vi "Main.vi"(8 "error in (no error)":errorcluster) -> ()   [LabVIEW 2017, in "FlagImpairModule.lvlib"]
uses:
  FlagImpairModule.lvlib
  <userlib>/NIST/ModuleAdminLib/ModuleAdmin/ModuleAdmin.lvclass
  C:/Program Files (x86)/National Instruments/LabVIEW 2017/user.lib/NIST/ModuleAdminLib/ModuleAdminBase/ModuleAdminBase.lvclass
  PublicAPI/Arguments/Requests/clStopArgument.ctl
  FlagImpairPlugins/FlagImpairPluginBase_class/FlagImpairPluginBase.lvclass
  C:/Program Files (x86)/National Instruments/LabVIEW 2017/user.lib/NIST/BaseClasses/BasePlugin_class/BasePlugin.lvclass
  <userlib>/NIST/ModuleAdminLib/ModuleAdmin/ModuleAdmin.lvclass/ModuleAdmin.ctl
  <userlib>/NIST/BaseClasses/BasePlugin_class/BasePlugin.lvclass/BasePlugin.ctl
  PublicAPI/Arguments/Requests/clFlagImpairConfig.ctl
  FlagImpairPlugins/FlagImpairPluginBase_class/TypeDefs/clFlagImpairConfig.ctl
  PublicAPI/Arguments/Requests/dblFlagImpairParams.ctl
  PublicAPI/Arguments/Requests/dblTimeArray.ctl
  <vilib>/Utility/error.llb/DialogType.ctl
  <userlib>/NIST/ModuleAdminLib/ModuleAdmin/Accessors/Read ShowPanel_.vi
  <userlib>/NIST/ModuleAdminLib/ModuleAdmin/Accessors/Write ShowPanel_.vi
  <userlib>/NIST/BaseClasses/BasePlugin_class/Accessors/Write PluginIniFilePath.vi
  <userlib>/NIST/BaseClasses/BasePlugin_class/Accessors/Read PluginIniFilePath.vi
  <userlib>/NIST/ModuleAdminLib/ModuleAdmin/Accessors/Read CloneRegRef.vi
  <vilib>/Utility/error.llb/Error Cluster From Error Code.vi
  FlagImpairPlugins/FlagImpairPluginBase_class/Accessors/Write clFlagImpairConfig.vi
  FlagImpairPlugins/FlagImpairPluginBase_class/Accessors/Read clFlagImpairConfig.vi
  FlagImpairPlugins/FlagImpairPluginBase_class/Accessors/Write FlagImpairParams.vi
  FlagImpairPlugins/FlagImpairPluginBase_class/Accessors/Read FlagImpairParams.vi
  FlagImpairPlugins/FlagImpairPluginBase_class/Accessors/Write TimeArray.vi
  FlagImpairPlugins/FlagImpairPluginBase_class/Accessors/Read TimeArray.vi
  FlagImpairPlugins/FlagImpairPluginBase_class/Accessors/Get FlagImpairmentArray.vi
  <vilib>/ErrorRing/Error Ring.xnode
  <userlib>/NIST/ModuleAdminLib/CloneRegistration/CloneRegistration.lvclass
  <userlib>/NIST/ModuleAdminLib/ModuleAdmin.lvlib
  <userlib>/NIST/BaseClasses/Object_class/BaseObject.lvclass
panel:
  out "error out":errorcluster
  in  "ModuleAdmin":refnum<class "ModuleAdmin.lvclass">
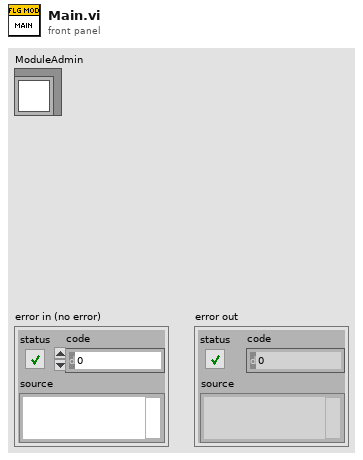
[diagram p1: front panel]
types:
  T1 = typedef "FlagImpairModule.lvlib/clRequestEvents.ctl" = cluster{"StopRequest":refnum<user-event>, "WriteFlagImpairConfigRequest":refnum<user-event>, "ReadFlagImpairConfigRequest":refnum<user-event>, "WriteFlagImpairParamsRequest":refnum<user-event>, "ReadFlagImpairParamsRequest":refnum<user-event>, "WriteTimeArrayRequest":refnum<user-event>, "ReadTimeArrayRequest":refnum<user-event>, "GetFlagImpairmentRequest":refnum<user-event>, "LoadPluginRequest":refnum<user-event>, "ReadPluginPathRequest":refnum<user-event>, "ShowPanelRequest":refnum<user-event>}
  T2 = typedef "FlagImpairModule.lvlib/clBroadcastEvents.ctl" = cluster{"DidInit":refnum<user-event>, "StatusUpdate":refnum<user-event>, "ErrorReport":refnum<user-event>, "DidStop":refnum<user-event>, "ReadFlagImpairConfig":refnum<user-event>, "ReadPluginINIFilePath":refnum<user-event>, "ReadFlagImpairParams":refnum<user-event>, "ReadTimeArray":refnum<user-event>, "GetFlagImpairment":refnum<user-event>}
  T3 = typedef "FlagImpairModule.lvlib/clStopArgument.ctl" = cluster{"Exit via Stop Module Req?":bool, "Wait for Module to stop?":bool, "ModuleAdmin":refnum<class "ModuleAdmin.lvclass">}
  T4 = enum32{"Invalid", "Standard", "Closed", "Hidden", "Minimized", "Maximized"}
  T5 = typedef "FlagImpairPlugins.lvlib/FlagImpairPluginBase.lvclass/clFlagImpairConfig.ctl" = cluster{"FlagImpairmentType":u16}
  T6 = typedef "FlagImpairModule.lvlib/clFlagImpairConfig.ctl" = cluster{"FlagImpairmentType":u16}
  T7 = typedef "FlagImpairModule.lvlib/dblFlagImpairParams.ctl" = dbl[][]
  T8 = typedef "FlagImpairModule.lvlib/dblTimeArray.ctl" = dbl[]
  T9 = typedef "FlagImpairPlugins.lvlib/FlagImpairPluginBase.lvclass/FlagImpairmentArray.ctl" = u32[]
  T10 = typedef "DialogType.ctl" = u16
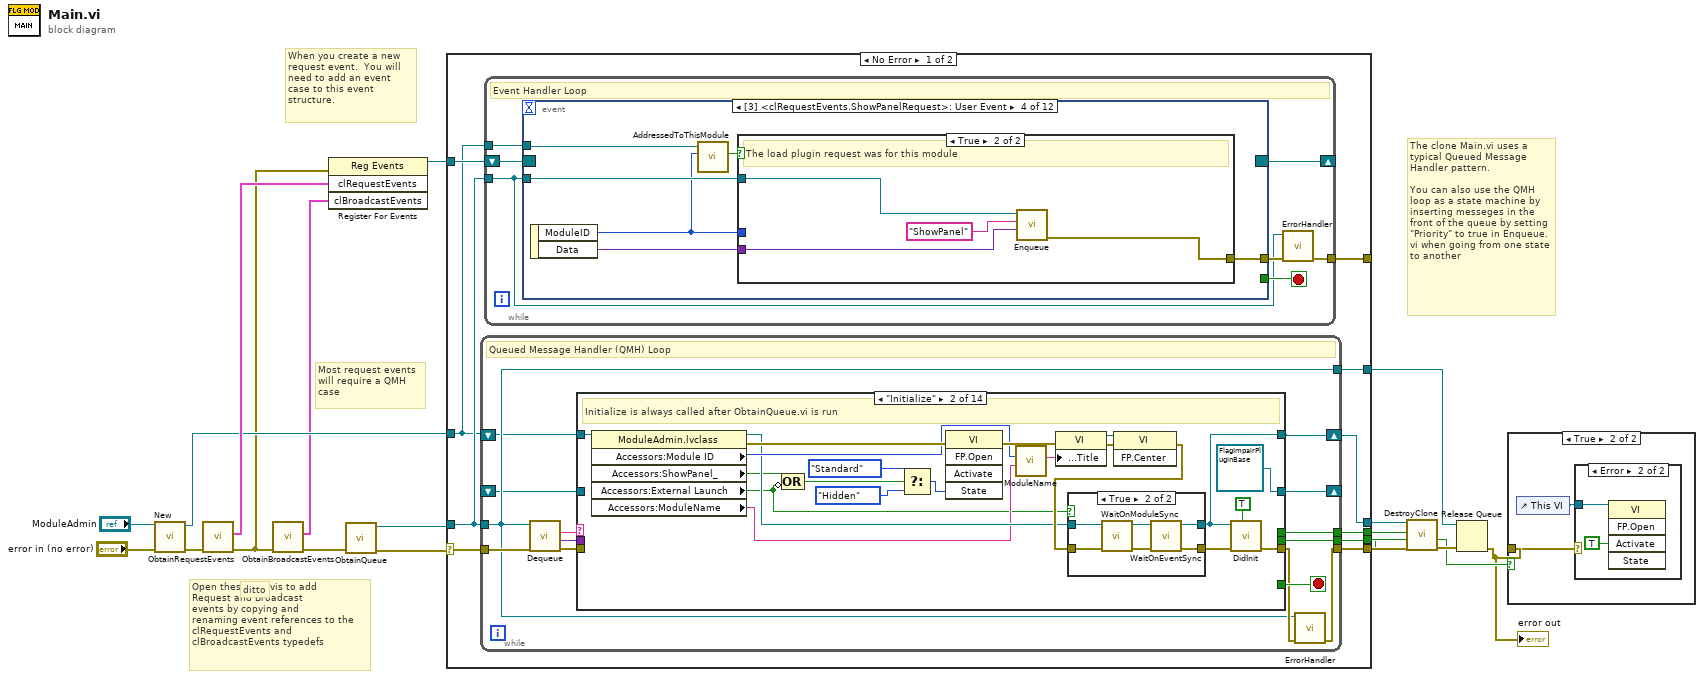
[diagram p0: block diagram]
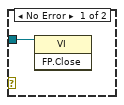
[diagram p3: hidden frame]
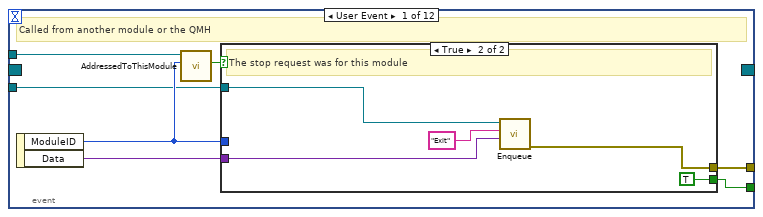
[diagram p4: hidden frame]
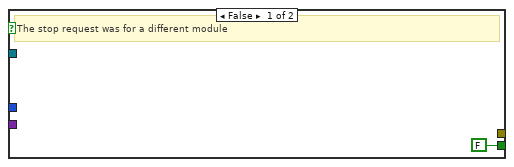
[diagram p5: hidden frame]
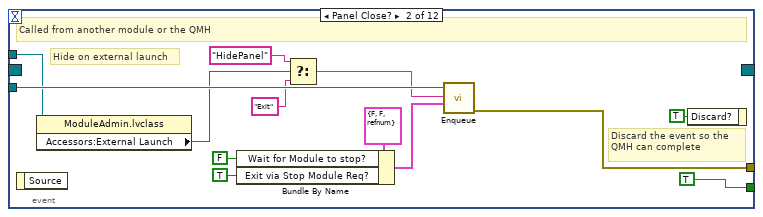
[diagram p6: hidden frame]
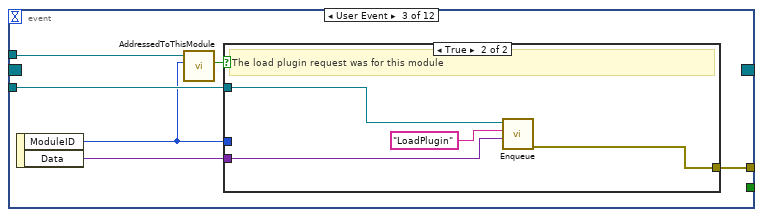
[diagram p7: hidden frame]
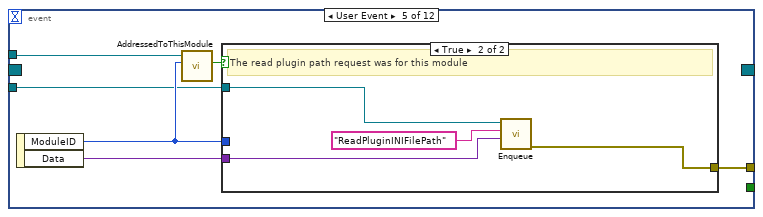
[diagram p10: hidden frame]
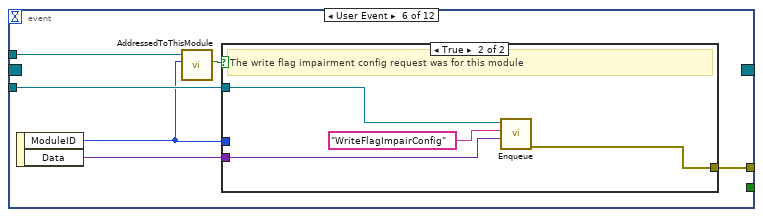
[diagram p12: hidden frame]
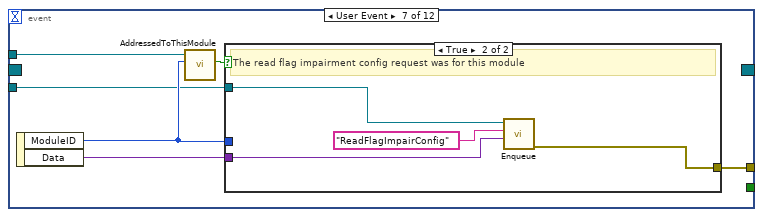
[diagram p14: hidden frame]
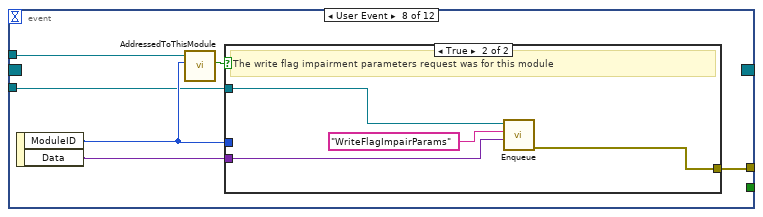
[diagram p16: hidden frame]
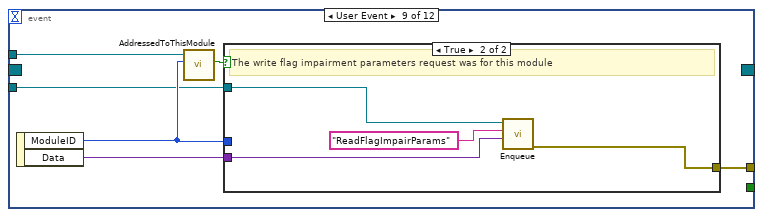
[diagram p18: hidden frame]
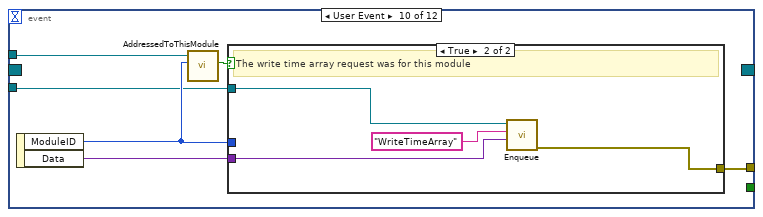
[diagram p20: hidden frame]
diagram:
  # "The clone Main.vi uses a typical Queued Message Handler pattern.  \n\nYou can also use the QMH loop as a state machine by inserting messeges in the front of the queue by setting \"Priority\" to true in Enqueue.vi when going from one state to another"
  # "Open these two vis to add\nRequest and Broadcast \nevents by copying and \nrenaming event references to the \nclRequestEvents and \nclBroadcastEvents typedefs"
  # "ditto"
  # "Most request events\nwill require a QMH\ncase"
  # "When you create a new request event.  You will need to add an event case to this event structure."
  n1 = call <userlib>:"New.vi"("error in (no error)"="error in (no error)", "ModuleAdmin"="ModuleAdmin") -> ("error out"=w17:errorcluster, "ModuleAdmin"=w13:refnum<class "ModuleAdmin.lvclass">)  [unwired: 7 in, 1 out]
  n2 = call "ObtainRequestEvents.vi"("error in (no error)"=w17) -> ("error out"=w10:errorcluster, "clRequestEvents"=w16:T1)  [unwired: 9 in]
  n3 = call "ObtainBroadcastEvents.vi"("error in (no error)"=w10) -> ("error out"=w11:errorcluster, "clBroadcastEvents"=w9:T2)  [unwired: 9 in]
  n4 = register-events(error in=w10, w16, w9) -> (reference out=w8:refnum<event-registration>)  [unwired: 1 in, 1 out]
  n5 = call "ObtainQueue.vi"("error in (no error)"=w11) -> ("error out"=w15:errorcluster, "MessageQueue"=w14:refnum<queue>)  [unwired: 9 in]
  n6 = case shown="No Error" w15 {
    selector: w15 -> [w29 w407]
    tunnel: w14 -> [w27 w403]
    tunnel: w13 -> [w24 w404]
    tunnel: [w28 w405] -> w7
    tunnel: [w26 w403] -> w12
    tunnel: w8 -> [w25 _]
    tunnel: [w23 w402] -> w5
    tunnel: [w22 _] -> w4
    tunnel: [w21 _] -> w3
    tunnel: [w20 _] -> _
    frame No Error {
      n7 = while {
        tunnel: w27 -> [w167]
        tunnel: w29 -> [w175]
        tunnel: [w169] -> w28
        tunnel: [w167] -> w26
        tunnel: [w171] -> w22
        tunnel: [w170] -> w21
        shift-right: [w166] -> _
        shift-left: _ -> [w165]
        shift-right: [w163] -> w23
        shift-left: w24 -> [w164]
        stop <- w176 stop-if-true
        # "Queued Message Handler (QMH) Loop"
        n8 = call "Dequeue.vi"("error in (no error)"=w175, "MessageQueue"=w167) -> ("error out"=w174:errorcluster, "Message Data"=w172:variant, "Message"=w173:string)  [unwired: 6 in, 1 out]
        n9 = case shown="\"Initialize\"" w173 {
          selector: w173 -> [w181 _ _ _ _ _ _ _ _ _ _ _ _ _]
          tunnel: [_ _ _ TRUE _ _ _ _ _ _ _ _ _ _] -> w176
          tunnel: w164 -> [w184 w213 w225 w234 w255 w264 w313 w331 w341 w353 w361 w372 w386 w398]
          tunnel: [w180 w202 w226 w241 w246 w269 w311 w327 w336 w349 w357 w370 w381 w396] -> w168
          tunnel: w174 -> [_ _ w227 w240 w254 w274 w321 w332 w339 w351 w360 w374 w389 w397]
          tunnel: w172 -> [_ _ w228 w239 w253 w273 w320 _ w338 _ w359 _ _ _]
          tunnel: [_ _ _ w237 _ _ _ _ _ _ _ _ _ _] -> w171
          tunnel: [_ _ _ w236 _ _ _ _ _ _ _ _ _ _] -> w170
          tunnel: [w178 refnum<class "FlagImpairPluginBase.lvclass"> refnum ("FlagImpairPlugins.lvlib:FlagImpairPluginBase.lvclass") w222 w235 w245 w268 w309 w323 w337 w350 w358 w371 w385 w393] -> w166
          tunnel: w165 -> [w178 _ w222 w235 w245 w272 w318 w333 w340 w352 w362 w373 w390 w399]
          tunnel: [w177 w193 w223 w234 w243 w262 w306 w322 w334 w347 w356 w369 w378 w391] -> w163
          frame Default {
            # "Called only if a message was queued and no QMH case was created"
            n10 = property class="ModuleAdmin.lvclass"(reference=w184) -> (reference out=w177:refnum<class "ModuleAdmin.lvclass">, "Accessors:Module ID"=w183:i32, "Accessors:ModuleName"=w179:string)  [unwired: 1 in, 1 out]
            n11 = call <userlib>:"ModuleName.vi"("Name"=w179, "ModuleID"=w183) -> ("ModuleName"=w182:string)  [unwired: 9 in]
            n12 = xnode "Error Ring"("parameter 0"=w181, "parameter 1"=w182) -> ("error out"=w180:errorcluster)
          }
          frame "Initialize" {
            # "Initialize is always called after ObtainQueue.vi is run"
            n13 = property class="ModuleAdmin.lvclass"(reference=w213) -> (reference out=w198:refnum<class "ModuleAdmin.lvclass">, error out=w210:errorcluster, "Accessors:Module ID"=w201:i32, "Accessors:ShowPanel_"=w196:bool, "Accessors:External Launch"=w195:bool, "Accessors:ModuleName"=w197:string)  [unwired: 1 in]
            n14 = Compound Arithmetic op=OR(w196, invert w195) -> (w194:bool)
            n15 = Select(t=T4."Standard" ("Front Panel Window:State"), s=w194, f=T4."Hidden" ("Front Panel Window:State")) -> (s? t:f=w206:T4)
            n16 = invoke class="VI" method="FP.Open"(error in=w210, "State"=w206) -> (error out=w209:errorcluster)  [unwired: 3 in, 4 out]
            n17 = call <userlib>:"ModuleName.vi"("Name"=w197, "ModuleID"=w201) -> ("ModuleName"=w205:string)  [unwired: 9 in]
            n18 = property class="VI"(error in=w209, "Front Panel.Title"=w205) -> (reference out=w212:refnum<vi>, error out=w211:errorcluster)  [unwired: 1 in]
            n19 = invoke class="VI" method="FP.Center"(reference=w212, error in=w211) -> (error out=w200:errorcluster)  [unwired: 1 in, 2 out]
            n20 = case shown="True" w195 {
              tunnel: [w215 w220] -> w203
              tunnel: [w214 w217] -> w193
              tunnel: w200 -> [w215 w219]
              tunnel: w198 -> [w214 w216]
              frame False {
              }
              frame True {
                n21 = call <userlib>:"WaitOnModuleSync.vi"("error in (no error)"=w219, "ModuleAdmin"=w216) -> ("error out"=w221:errorcluster, "ModuleAdmin"=w218:refnum<class "ModuleAdmin.lvclass">)  [unwired: 8 in]
                n22 = call <userlib>:"WaitOnEventSync.vi"("error in (no error)"=w221, "ModuleAdmin"=w218) -> ("error out"=w220:errorcluster, "ModuleAdmin"=w217:refnum<class "ModuleAdmin.lvclass">)  [unwired: 8 in]
              }
            }
            n23 = call "DidInit.vi"("Init?"=TRUE, "error in (no error)"=w203, "ModuleAdmin"=w193) -> ("error out"=w202:errorcluster)  [unwired: 8 in]
          }
          frame "ShowPanel" {
            n24 = Variant To Data(error in=w227, type=FALSE, Variant=w228) -> (data=w224:bool, error out=w230:errorcluster)
            n25 = Select(t=T4."Standard" ("Front Panel Window:State"), s=w224, f=T4."Hidden" ("Front Panel Window:State")) -> (s? t:f=w233:T4)
            n26 = property class="VI"(error in=w230, "FP.State"=w233) -> (error out=w226:errorcluster)  [unwired: 1 in, 1 out]
            n27 = property class="ModuleAdmin.lvclass"(reference=w225, "Accessors:ShowPanel_"=w224) -> (reference out=w223:refnum<class "ModuleAdmin.lvclass">)  [unwired: 1 in, 1 out]
          }
          frame "Exit" {
            # "Called by the StopRequest event handler case"
            n28 = control-ref of="This VI"() -> (w238:refnum<vi>)
            n29 = call "HandleExit.vi"("error in (no error)"=w240, "VI Refnum"=w238, "StopArgument"=w239, "ModuleAdmin"=w234) -> ("error out"=w241:errorcluster, "Exit via Stop Module Req?"=w236:bool, "WaitForStop?"=w237:bool)  [unwired: 5 in]
          }
          frame "Error" {
            n30 = property class="ModuleAdmin.lvclass"(reference=w255) -> (reference out=w244:refnum<class "ModuleAdmin.lvclass">, "Accessors:External Launch"=w249:bool, "Accessors:Module ID"=w247:i32)  [unwired: 1 in, 1 out]
            n31 = Variant To Data(error in=w254, type=errorcluster {"status"=FALSE, "code"=0, "source"=""} ("error constant"), Variant=w253) -> (data=w248:errorcluster, error out=w251:errorcluster)
            n32 = call "ReportError.vi"("error in (no error)"=w251, "ErrorReported"=w248, "ModuleID"=w247) -> ("error out"=w250:errorcluster)  [unwired: 8 in]
            n33 = case shown="False" w249 {
              tunnel: w250 -> [w259 w261]
              tunnel: w248 -> [w258 _]
              tunnel: [w257 w261] -> w246
              tunnel: w244 -> [w256 w260]
              tunnel: [w256 w260] -> w243
              frame False {
                # "Todo:  Add an event to ask the user\nIf the module should stop or continue"
                # "Stand alone: now, force an exit"
                n34 = call <vilib>:"Simple Error Handler.vi"("error in (no error)"=w258) -> ()  [unwired: 4 in, 5 out]
                n35 = call "StopRequest.vi"("error in (no error)"=w259, "ModuleAdmin"=w256) -> ("error out"=w257:errorcluster)  [unwired: 8 in, 1 out]
              }
              frame True {
                # "Externally launched modules only broadcast the error msg"
              }
            }
          }
          frame "LoadPlugin" {
            # "Load the plugin specified from the INI file.  Save the INI file path in the plugin class."
            n36 = Variant To Data(error in=w274, type=path "", Variant=w273) -> (data=w263:path, error out=w278:errorcluster)
            n37 = call <userlib>:"GetPathToClass.vi"("error in (no error)"=w278, "configuration file path"=w263) -> ("error IO"=w277:errorcluster, "PathToClass"=w265:path)  [unwired: 8 in]
            n38 = Current VI's Path() -> (path=w266:path)
            n39 = Build Path(base path=w266, name or relative path=w265) -> (appended path=w267:path)
            n40 = call <vilib>:"Check if File or Folder Exists.vi"("error in (no error)"=w277, "path"=w267) -> ("error out"=w275:errorcluster, "file or folder exists?"=w276:bool, "dup path"=w271:path)  [unwired: 7 in]
            n41 = case shown="False" w276 {
              tunnel: w271 -> [w283 w293]
              tunnel: w275 -> [w291 w298]
              tunnel: [w286 w296] -> w269
              tunnel: [w284 w297] -> w270
              tunnel: w272 -> [_ w297]
              tunnel: w264 -> [w282 w292]
              tunnel: [w280 w292] -> w262
              frame True {
                n42 = property class="ModuleAdmin.lvclass"(reference=w282) -> (reference out=w280:refnum<class "ModuleAdmin.lvclass">, "Accessors:Module ID"=w281:i32)  [unwired: 1 in, 1 out]
                n43 = call-dynamic "LoadClassFromFile.vi"("error in (no error)"=w291, "class path"=w283, "reference in"=refnum<class "FlagImpairPluginBase.lvclass"> refnum ("FlagImpairPlugins.lvlib:FlagImpairPluginBase.lvclass")) -> ("error out"=w285:errorcluster, "reference out"=w284:refnum<class "FlagImpairPluginBase.lvclass">)  [unwired: 7 in]
                n44 = Path To String(path=w283) -> (string=w287:string)
                n45 = Format Into String(format string="Plugin %s loaded", w287) -> (resulting string=w288:string)  [unwired: 2 in, 1 out]
                n46 = call "StatusUpdate.vi"("error in (no error)"=w285, "Status"=w288, "ModuleID"=w281) -> ("error out"=w286:errorcluster)  [unwired: 8 in]
              }
              frame False {
                n47 = Path To String(path=w293) -> (string=w294:string)
                n48 = xnode "Error Ring"("parameter 0"=w294) -> ("error out"=w295:errorcluster)
                n49 = Merge Errors(w295, w298) -> (w296:errorcluster)
              }
            }
            n50 = property class="FlagImpairPluginBase.lvclass"(reference=w270, "Accessors:PluginIniFilePath"=w263) -> (reference out=w268:refnum<class "FlagImpairPluginBase.lvclass">)  [unwired: 1 in, 1 out]
          }
          frame "WriteFlagImpairConfig" {
            # "Write the flag impairment config cluster to the plugin class and send a status update."
            n51 = Variant To Data(error in=w321, type=T6 {"FlagImpairmentType"=0} ("clFlagImpairConfig"), Variant=w320) -> (data=w316:T6, error out=w312:errorcluster)
            n52 = Unbundle By Name(w316) -> ("FlagImpairmentType"=w314:u16)
            n53 = Bundle By Name(cluster=T5 {"FlagImpairmentType"=0} ("clFlagImpairConfig"), "FlagImpairmentType"=w314) -> (w315:T5)
            n54 = property class="FlagImpairPluginBase.lvclass"(reference=w318, error in=w312, "Accessors:clFlagImpairConfig"=w315) -> (reference out=w309:refnum<class "FlagImpairPluginBase.lvclass">, error out=w308:errorcluster)
            n55 = property class="ModuleAdmin.lvclass"(reference=w313) -> (reference out=w306:refnum<class "ModuleAdmin.lvclass">, "Accessors:Module ID"=w310:i32)  [unwired: 1 in, 1 out]
            n56 = call "StatusUpdate.vi"("error in (no error)"=w308, "Status"="Config Received", "ModuleID"=w310) -> ("error out"=w311:errorcluster)  [unwired: 8 in]
          }
          frame "ReadFlagImpairConfig" {
            # "Broadcast the flag impairment configuration."
            n57 = property class="FlagImpairPluginBase.lvclass"(reference=w333, error in=w332) -> (reference out=w323:refnum<class "FlagImpairPluginBase.lvclass">, error out=w324:errorcluster, "Accessors:clFlagImpairConfig"=w330:T5)
            n58 = Unbundle By Name(w330) -> ("FlagImpairmentType"=w329:u16)
            n59 = Bundle By Name(cluster=T6 {"FlagImpairmentType"=0} ("clFlagImpairConfig"), "FlagImpairmentType"=w329) -> (w325:T6)
            n60 = property class="ModuleAdmin.lvclass"(reference=w331) -> (reference out=w322:refnum<class "ModuleAdmin.lvclass">, "Accessors:Module ID"=w326:i32)  [unwired: 1 in, 1 out]
            n61 = call "ReadFlagImpairConfig.vi"("error in (no error)"=w324, "clFlagImpairConfig"=w325, "ModuleID"=w326) -> ("error out"=w327:errorcluster)  [unwired: 8 in]
          }
          frame "WriteFlagImpairParams" {
            w346 = T7 []  # dblFlagImpairParams
            # "Write the flag impairment parameters to the plugin class."
            n62 = Variant To Data(error in=w339, type=w346, Variant=w338) -> (data=w335:T7, error out=w345:errorcluster)
            n63 = property class="FlagImpairPluginBase.lvclass"(reference=w340, error in=w345, "Accessors:dblFlagImpairParams"=w335) -> (reference out=w337:refnum<class "FlagImpairPluginBase.lvclass">, error out=w343:errorcluster)
            n64 = property class="ModuleAdmin.lvclass"(reference=w341) -> (reference out=w334:refnum<class "ModuleAdmin.lvclass">, "Accessors:Module ID"=w344:i32)  [unwired: 1 in, 1 out]
            n65 = call "StatusUpdate.vi"("error in (no error)"=w343, "Status"="Params Received", "ModuleID"=w344) -> ("error out"=w336:errorcluster)  [unwired: 8 in]
          }
          frame "ReadFlagImpairParams" {
            # "Broadcast the flag impairment parameters."
            n66 = property class="FlagImpairPluginBase.lvclass"(reference=w352, error in=w351) -> (reference out=w350:refnum<class "FlagImpairPluginBase.lvclass">, error out=w354:errorcluster, "Accessors:dblFlagImpairParams"=w348:dbl[][])
            n67 = property class="ModuleAdmin.lvclass"(reference=w353) -> (reference out=w347:refnum<class "ModuleAdmin.lvclass">, "Accessors:Module ID"=w355:i32)  [unwired: 1 in, 1 out]
            n68 = call "ReadFlagImpairParams.vi"("error in (no error)"=w354, "clFlagImpairParams"=w348, "ModuleID"=w355) -> ("error out"=w349:errorcluster)  [unwired: 8 in]
          }
          frame "WriteTimeArray" {
            w368 = T8 []  # dblTimeArray
            # "Write the time array to the plugin class."
            n69 = Variant To Data(error in=w360, type=w368, Variant=w359) -> (data=w363:T8, error out=w367:errorcluster)
            n70 = property class="FlagImpairPluginBase.lvclass"(reference=w362, error in=w367, "Accessors:dblTimeArray"=w363) -> (reference out=w358:refnum<class "FlagImpairPluginBase.lvclass">, error out=w365:errorcluster)
            n71 = property class="ModuleAdmin.lvclass"(reference=w361) -> (reference out=w356:refnum<class "ModuleAdmin.lvclass">, "Accessors:Module ID"=w366:i32)  [unwired: 1 in, 1 out]
            n72 = call "StatusUpdate.vi"("error in (no error)"=w365, "Status"="Time Array Received", "ModuleID"=w366) -> ("error out"=w357:errorcluster)  [unwired: 8 in]
          }
          frame "ReadTimeArray" {
            # "Broadcast the time array from the flag impairment module."
            n73 = property class="FlagImpairPluginBase.lvclass"(reference=w373, error in=w374) -> (reference out=w371:refnum<class "FlagImpairPluginBase.lvclass">, error out=w376:errorcluster, "Accessors:dblTimeArray"=w375:dbl[])
            n74 = property class="ModuleAdmin.lvclass"(reference=w372) -> (reference out=w369:refnum<class "ModuleAdmin.lvclass">, "Accessors:Module ID"=w377:i32)  [unwired: 1 in, 1 out]
            n75 = call "ReadTimeArray.vi"("error in (no error)"=w376, "dblTimeArray"=w375, "ModuleID"=w377) -> ("error out"=w370:errorcluster)  [unwired: 8 in]
          }
          frame "GetFlagImpairment" {
            # "Get the flag impairment data and broadcast the flag impairment array."
            n76 = call-dynamic "GetFlags.vi"("error in (no error)"=w389, "FlagImpairPluginBase in"=w390) -> ("error out"=w387:errorcluster, "FlagImpairPluginBase out"=w388:refnum<class "FlagImpairPluginBase.lvclass">)  [unwired: 8 in]
            n77 = property class="FlagImpairPluginBase.lvclass"(reference=w388, error in=w387) -> (reference out=w385:refnum<class "FlagImpairPluginBase.lvclass">, error out=w384:errorcluster, "Accessors:u32FlagImpairmentArray"=w383:T9)
            n78 = property class="ModuleAdmin.lvclass"(reference=w386) -> (reference out=w378:refnum<class "ModuleAdmin.lvclass">, "Accessors:Module ID"=w380:i32)  [unwired: 1 in, 1 out]
            n79 = call "GetFlagImpairmentArray.vi"("error in (no error)"=w384, "ui32FlagImpairmentArray"=w383, "ModuleID"=w380) -> ("error out"=w382:errorcluster)  [unwired: 8 in]
            n80 = call "StatusUpdate.vi"("error in (no error)"=w382, "Status"="Impairment Transmitted", "ModuleID"=w380) -> ("error out"=w381:errorcluster)  [unwired: 8 in]
          }
          frame "ReadPluginINIFilePath" {
            # "Read the plugin INI file path from the plugin class and broadcast the path."
            n81 = property class="FlagImpairPluginBase.lvclass"(reference=w399, error in=w397) -> (reference out=w393:refnum<class "FlagImpairPluginBase.lvclass">, error out=w395:errorcluster, "Accessors:PluginIniFilePath"=w392:path)
            n82 = property class="ModuleAdmin.lvclass"(reference=w398) -> (reference out=w391:refnum<class "ModuleAdmin.lvclass">, "Accessors:Module ID"=w394:i32)  [unwired: 1 in, 1 out]
            n83 = call "ReadPluginINIFilePath.vi"("error in (no error)"=w395, "Path"=w392, "ModuleID"=w394) -> ("error out"=w396:errorcluster)  [unwired: 8 in]
          }
        }
        n84 = call "ErrorHandler.vi"("error in (no error)"=w168, "MessageQueue"=w167) -> ("error out"=w169:errorcluster)  [unwired: 8 in, 1 out]
      }
      n85 = while {
        tunnel: w27 -> [w30]
        shift-right: [w34] -> _
        shift-left: w25 -> [w35]
        tunnel: w24 -> [w33]
        tunnel: [w31] -> w20
        stop <- w36 stop-if-true
        # "Event Handler Loop"
        n86 = event shown="[3] <clRequestEvents.ShowPanelRequest>: User Event" {
          selector: w35 -> [_ _ _ _ _ _ _ _ _ _ _ _]
          dyn-events: [_ _ _ _ _ _ _ _ _ _ _ _] -> w34
          timeout: _ -> [_ _ _ _ _ _ _ _ _ _ _ _]
          tunnel: w30 -> [w40 w62 w67 w77 w85 w97 w105 w115 w125 w135 w144 w157]
          tunnel: [w39 TRUE _ _ _ _ _ _ _ _ _ _] -> w36
          tunnel: w33 -> [w43 w56 w66 w76 w84 w96 w104 w114 w124 w134 w143 w156]
          tunnel: [w38 w60 w63 w73 w83 w93 w103 w113 w123 w133 w147 w153] -> w32
          event User Event {
            # "Called from another module or the QMH"
            n87 = event-data() -> ("ModuleID"=w41:i32, "Data"=w37:variant)  [unwired: 1 in]
            n88 = call <userlib>:"AddressedToThisModule.vi"("ModuleID"=w41, "ModuleAdmin"=w43) -> ("AddressedToThisInstance?"=w42:bool)  [unwired: 8 in, 1 out]
            n89 = case shown="True" w42 {
              tunnel: w41 -> [_ _]
              tunnel: w40 -> [_ w49]
              tunnel: [FALSE TRUE] -> w39
              tunnel: [_ w47] -> w38
              tunnel: w37 -> [_ w45]
              frame False {
                # "The stop request was for a different module"
              }
              frame True {
                # "The stop request was for this module"
                n90 = call "Enqueue.vi"("Message Data"=w45, "Message"="Exit", "MessageQueue"=w49) -> ("error out"=w47:errorcluster)  [unwired: 7 in, 1 out]
              }
            }
          }
          event Panel Close? {
            # "Hide on external launch"
            # "Discard the event so the QMH can complete"
            # "Called from another module or the QMH"
            n91 = event-data() -> ()  [unwired: 1 in, 1 out]
            n92 = property class="ModuleAdmin.lvclass"(reference=w56) -> ("Accessors:External Launch"=w51:bool)  [unwired: 1 in, 2 out]
            n93 = Bundle By Name(cluster=T3 {"Exit via Stop Module Req?"=FALSE, "Wait for Module to stop?"=FALSE, "ModuleAdmin"=refnum} ("Stop Argument"), "Wait for Module to stop?"=FALSE, "Exit via Stop Module Req?"=TRUE) -> (w57:T3)
            n94 = Select(t="HidePanel", s=w51, f="Exit" ("Message")) -> (s? t:f=w53:string)
            n95 = call "Enqueue.vi"("Message Data"=w57, "Message"=w53, "MessageQueue"=w62) -> ("error out"=w60:errorcluster)  [unwired: 7 in, 1 out]
            n96 = event-data("Discard?"=TRUE) -> ()  [unwired: 1 in, 1 out]
          }
          event User Event {
            n97 = event-data() -> ("ModuleID"=w65:i32, "Data"=w64:variant)  [unwired: 1 in]
            n98 = call <userlib>:"AddressedToThisModule.vi"("ModuleID"=w65, "ModuleAdmin"=w66) -> ("AddressedToThisInstance?"=w68:bool)  [unwired: 8 in, 1 out]
            n99 = case shown="True" w68 {
              tunnel: w65 -> [_ _]
              tunnel: w67 -> [_ w72]
              tunnel: [_ w71] -> w63
              tunnel: w64 -> [_ w69]
              frame False {
                # "The stop request was for a different module"
              }
              frame True {
                # "The load plugin request was for this module"
                n100 = call "Enqueue.vi"("Message Data"=w69, "Message"="LoadPlugin", "MessageQueue"=w72) -> ("error out"=w71:errorcluster)  [unwired: 7 in, 1 out]
              }
            }
          }
          event User Event {
            n101 = event-data() -> ("ModuleID"=w75:i32, "Data"=w74:variant)  [unwired: 1 in]
            n102 = call <userlib>:"AddressedToThisModule.vi"("ModuleID"=w75, "ModuleAdmin"=w76) -> ("AddressedToThisInstance?"=w78:bool)  [unwired: 8 in, 1 out]
            n103 = case shown="True" w78 {
              tunnel: w75 -> [_ _]
              tunnel: w77 -> [_ w82]
              tunnel: [_ w81] -> w73
              tunnel: w74 -> [_ w79]
              frame False {
                # "The stop request was for a different module"
              }
              frame True {
                # "The load plugin request was for this module"
                n104 = call "Enqueue.vi"("Message Data"=w79, "Message"="ShowPanel", "MessageQueue"=w82) -> ("error out"=w81:errorcluster)  [unwired: 7 in, 1 out]
              }
            }
          }
          event User Event {
            n105 = event-data() -> ("ModuleID"=w87:i32, "Data"=w86:variant)  [unwired: 1 in]
            n106 = call <userlib>:"AddressedToThisModule.vi"("ModuleID"=w87, "ModuleAdmin"=w84) -> ("AddressedToThisInstance?"=w88:bool)  [unwired: 8 in, 1 out]
            n107 = case shown="True" w88 {
              tunnel: w87 -> [_ _]
              tunnel: w85 -> [_ w92]
              tunnel: [_ w91] -> w83
              tunnel: w86 -> [_ w89]
              frame False {
                # "The stop request was for a different module"
              }
              frame True {
                # "The read plugin path request was for this module"
                n108 = call "Enqueue.vi"("Message Data"=w89, "Message"="ReadPluginINIFilePath", "MessageQueue"=w92) -> ("error out"=w91:errorcluster)  [unwired: 7 in, 1 out]
              }
            }
          }
          event User Event {
            n109 = event-data() -> ("ModuleID"=w95:i32, "Data"=w94:variant)  [unwired: 1 in]
            n110 = call <userlib>:"AddressedToThisModule.vi"("ModuleID"=w95, "ModuleAdmin"=w96) -> ("AddressedToThisInstance?"=w98:bool)  [unwired: 8 in, 1 out]
            n111 = case shown="True" w98 {
              tunnel: w95 -> [_ _]
              tunnel: w97 -> [_ w102]
              tunnel: [_ w101] -> w93
              tunnel: w94 -> [_ w99]
              frame False {
                # "The stop request was for a different module"
              }
              frame True {
                # "The write flag impairment config request was for this module"
                n112 = call "Enqueue.vi"("Message Data"=w99, "Message"="WriteFlagImpairConfig", "MessageQueue"=w102) -> ("error out"=w101:errorcluster)  [unwired: 7 in, 1 out]
              }
            }
          }
          event User Event {
            n113 = event-data() -> ("ModuleID"=w107:i32, "Data"=w106:variant)  [unwired: 1 in]
            n114 = call <userlib>:"AddressedToThisModule.vi"("ModuleID"=w107, "ModuleAdmin"=w104) -> ("AddressedToThisInstance?"=w108:bool)  [unwired: 8 in, 1 out]
            n115 = case shown="True" w108 {
              tunnel: w107 -> [_ _]
              tunnel: w105 -> [_ w112]
              tunnel: [_ w111] -> w103
              tunnel: w106 -> [_ w109]
              frame False {
                # "The stop request was for a different module"
              }
              frame True {
                # "The read flag impairment config request was for this module"
                n116 = call "Enqueue.vi"("Message Data"=w109, "Message"="ReadFlagImpairConfig", "MessageQueue"=w112) -> ("error out"=w111:errorcluster)  [unwired: 7 in, 1 out]
              }
            }
          }
          event User Event {
            n117 = event-data() -> ("ModuleID"=w116:i32, "Data"=w117:variant)  [unwired: 1 in]
            n118 = call <userlib>:"AddressedToThisModule.vi"("ModuleID"=w116, "ModuleAdmin"=w114) -> ("AddressedToThisInstance?"=w118:bool)  [unwired: 8 in, 1 out]
            n119 = case shown="True" w118 {
              tunnel: w116 -> [_ _]
              tunnel: w115 -> [_ w122]
              tunnel: [_ w121] -> w113
              tunnel: w117 -> [_ w119]
              frame False {
                # "The stop request was for a different module"
              }
              frame True {
                # "The write flag impairment parameters request was for this module"
                n120 = call "Enqueue.vi"("Message Data"=w119, "Message"="WriteFlagImpairParams", "MessageQueue"=w122) -> ("error out"=w121:errorcluster)  [unwired: 7 in, 1 out]
              }
            }
          }
          event User Event {
            n121 = event-data() -> ("ModuleID"=w127:i32, "Data"=w126:variant)  [unwired: 1 in]
            n122 = call <userlib>:"AddressedToThisModule.vi"("ModuleID"=w127, "ModuleAdmin"=w124) -> ("AddressedToThisInstance?"=w128:bool)  [unwired: 8 in, 1 out]
            n123 = case shown="True" w128 {
              tunnel: w127 -> [_ _]
              tunnel: w125 -> [_ w132]
              tunnel: [_ w131] -> w123
              tunnel: w126 -> [_ w129]
              frame False {
                # "The stop request was for a different module"
              }
              frame True {
                # "The write flag impairment parameters request was for this module"
                n124 = call "Enqueue.vi"("Message Data"=w129, "Message"="ReadFlagImpairParams", "MessageQueue"=w132) -> ("error out"=w131:errorcluster)  [unwired: 7 in, 1 out]
              }
            }
          }
          event User Event {
            n125 = event-data() -> ("ModuleID"=w137:i32, "Data"=w136:variant)  [unwired: 1 in]
            n126 = call <userlib>:"AddressedToThisModule.vi"("ModuleID"=w137, "ModuleAdmin"=w134) -> ("AddressedToThisInstance?"=w138:bool)  [unwired: 8 in, 1 out]
            n127 = case shown="True" w138 {
              tunnel: w137 -> [_ _]
              tunnel: w135 -> [_ w142]
              tunnel: [_ w141] -> w133
              tunnel: w136 -> [_ w139]
              frame False {
                # "The stop request was for a different module"
              }
              frame True {
                # "The write time array request was for this module"
                n128 = call "Enqueue.vi"("Message Data"=w139, "Message"="WriteTimeArray", "MessageQueue"=w142) -> ("error out"=w141:errorcluster)  [unwired: 7 in, 1 out]
              }
            }
          }
          event User Event {
            n129 = event-data() -> ("ModuleID"=w145:i32, "Data"=w146:variant)  [unwired: 1 in]
            n130 = call <userlib>:"AddressedToThisModule.vi"("ModuleID"=w145, "ModuleAdmin"=w143) -> ("AddressedToThisInstance?"=w148:bool)  [unwired: 8 in, 1 out]
            n131 = case shown="True" w148 {
              tunnel: w145 -> [_ _]
              tunnel: w144 -> [_ w152]
              tunnel: [_ w151] -> w147
              tunnel: w146 -> [_ w149]
              frame False {
                # "The stop request was for a different module"
              }
              frame True {
                # "The read time array request was for this module"
                n132 = call "Enqueue.vi"("Message Data"=w149, "Message"="ReadTimeArray", "MessageQueue"=w152) -> ("error out"=w151:errorcluster)  [unwired: 7 in, 1 out]
              }
            }
          }
          event User Event {
            n133 = event-data() -> ("ModuleID"=w155:i32, "Data"=w154:variant)  [unwired: 1 in]
            n134 = call <userlib>:"AddressedToThisModule.vi"("ModuleID"=w155, "ModuleAdmin"=w156) -> ("AddressedToThisInstance?"=w158:bool)  [unwired: 8 in, 1 out]
            n135 = case shown="True" w158 {
              tunnel: w155 -> [_ _]
              tunnel: w157 -> [_ w162]
              tunnel: [_ w161] -> w153
              tunnel: w154 -> [_ w159]
              frame False {
                # "The stop request was for a different module"
              }
              frame True {
                # "The get flag impairment request was for this module"
                n136 = call "Enqueue.vi"("Message Data"=w159, "Message"="GetFlagImpairment", "MessageQueue"=w162) -> ("error out"=w161:errorcluster)  [unwired: 7 in, 1 out]
              }
            }
          }
        }
        n137 = call "ErrorHandler.vi"("error in (no error)"=w32, "MessageQueue"=w30) -> ("error out"=w31:errorcluster)  [unwired: 8 in, 1 out]
      }
    }
    frame Error {
      n138 = property class="ModuleAdmin.lvclass"(reference=w404) -> (reference out=w402:refnum<class "ModuleAdmin.lvclass">, "Accessors:CloneRegRef"=w401:refnum<data-value>, "Accessors:Module ID"=w400:i32)  [unwired: 1 in, 1 out]
      n139 = call <userlib>:"Remove.vi"("Module ID"=w400, "CloneRegRef"=w401) -> ("error out"=w406:errorcluster)  [unwired: 7 in, 2 out]
      n140 = flat-sequence {
        tunnel: w407 -> [w410]
        tunnel: w406 -> [_]
        tunnel: [w408] -> w405
        frame #0 {
          w409 = T10 2 items=["no dialog", "OK message", "continue or stop message", "OK message + warnings", "continue/stop + warnings"] ("type of dialog (OK msg:1)")
          n141 = call <vilib>:"Simple Error Handler.vi"("type of dialog (OK msg:1)"=w409, "error in (no error)"=w410) -> ("error out"=w408:errorcluster)  [unwired: 3 in, 4 out]
        }
      }
    }
  }
  n142 = call "DestroyClone.vi"("error in (no error)"=w7, "Exit via Stop Module Req?"=w3, "Wait for Module to stop?"=w4, "ModuleAdmin"=w5) -> ("error out"=w6:errorcluster, "External Launch"=w2:bool)  [unwired: 5 in, 1 out]
  n143 = Release Queue(queue=w12, error in (no error)=w6) -> (error out=w1:errorcluster)  [unwired: 1 in, 2 out]
  "error out" <- w1
  n144 = case shown="True" w2 {
    tunnel: w1 -> [_ w412]
    frame False {
    }
    frame True {
      n145 = control-ref of="This VI"() -> (w411:refnum<vi>)
      n146 = case shown="Error" w412 {
        tunnel: w411 -> [w413 w414]
        frame No Error {
          n147 = invoke class="VI" method="FP.Close"(reference=w413) -> ()  [unwired: 2 in, 3 out]
        }
        frame Error {
          n148 = invoke class="VI" method="FP.Open"(reference=w414, "Activate"=TRUE ("Activate?")) -> ()  [unwired: 3 in, 5 out]
        }
      }
    }
  }
